vi "Byte_Generator.vi"(0 "Data_In":T1, 5 "Byte_Array":dbl[](array[numeric])) -> (4 "Data_Out":T1)   [LabVIEW 2023]
uses:
  Controls/Byte_Generator_Data.ctl
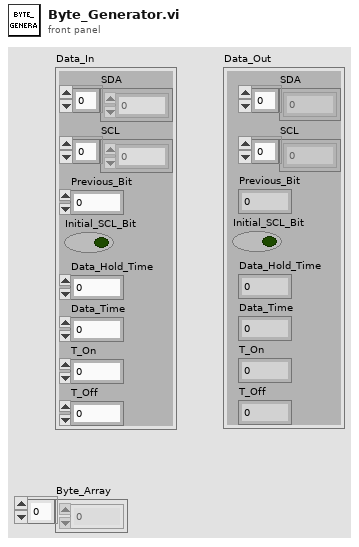
[diagram p1: front panel]
types:
  T1 = typedef "Byte_Generator_Data.ctl" = cluster{"SDA":dbl[], "SCL":dbl[], "Previous_Bit":dbl, "Initial_SCL_Bit":bool, "Data_Hold_Time":i32, "Data_Time":i32, "T_On":i32, "T_Off":i32}
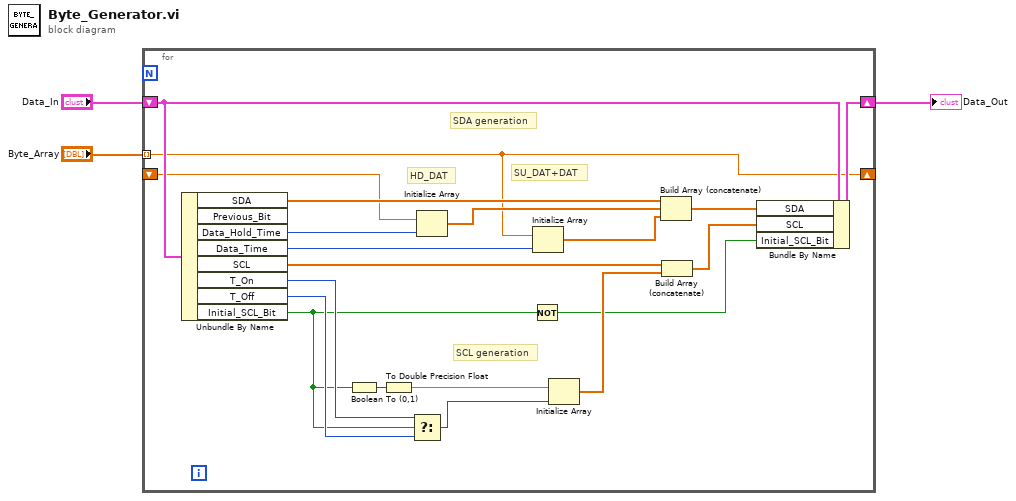
[diagram p0: block diagram]
diagram:
  n1 = for {
    shift-right: [w17] -> w2
    shift-left: "Data_In" -> [w18]
    tunnel: "Byte_Array" -> [w5] mode=indexing
    shift-right: [w5] -> _
    shift-left: _ -> [w4]
    # "HD_DAT"
    # "SDA generation"
    # "SCL generation"
    # "SU_DAT+DAT"
    n2 = Unbundle By Name(w18) -> ("SDA"=w19:dbl[], "Data_Hold_Time"=w11:i32, "Data_Time"=w10:i32, "SCL"=w6:dbl[], "T_On"=w9:i32, "T_Off"=w8:i32, "Initial_SCL_Bit"=w7:bool)  [unwired: 1 out]
    n3 = Boolean To (0,1)(Boolean=w7) -> (0, 1=w23:i16)
    n4 = To Double Precision Float(number=w23) -> (double precision float=w22:dbl)
    n5 = Select(t=w9, s=w7, f=w8) -> (s? t:f=w21:i32)
    n6 = Initialize Array(w4, w11) -> (w12:dbl[])
    n7 = Not(x=w7) -> (.not. x?=w14:bool)
    n8 = Initialize Array(w5, w10) -> (w13:dbl[])
    n9 = Initialize Array(w22, w21) -> (w20:dbl[])
    n10 = Build Array (concatenate)(w19, w12, w13) -> (w16:dbl[])
    n11 = Build Array (concatenate)(w6, w20) -> (w15:dbl[])
    n12 = Bundle By Name(cluster=w18, "SDA"=w16, "SCL"=w15, "Initial_SCL_Bit"=w14) -> (w17:T1)
  }
  "Data_Out" <- w2
